vi "ClearDataContainer.vi"(8 "error in (no error)":errorcluster, 11 "Task_Abstr in":refnum<class "Task_Abstr.lvclass">) -> (0 "error out":errorcluster, 3 "Task_Abstr out":refnum<class "Task_Abstr.lvclass">)   [LabVIEW 2025, in "Task_Abstr.lvlib" / "Task_Abstr.lvclass"]
uses:
  Task_Abstr.lvclass
  DataContainer.ctl
  WaveformData.ctl
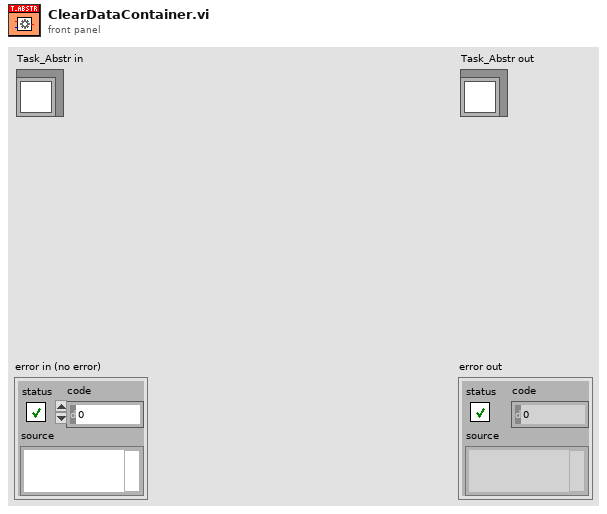
[diagram p1: front panel]
types:
  T1 = typedef "Task_Abstr.lvlib/Task_Abstr.lvclass/DataContainer.ctl" = map{string, T2}
  T2 = typedef "Task_Abstr.lvlib/Task_Abstr.lvclass/WaveformData.ctl" = cluster{"StartTime":timestamp, "StopTime":timestamp, "Waveform":waveform(dbl)[]}
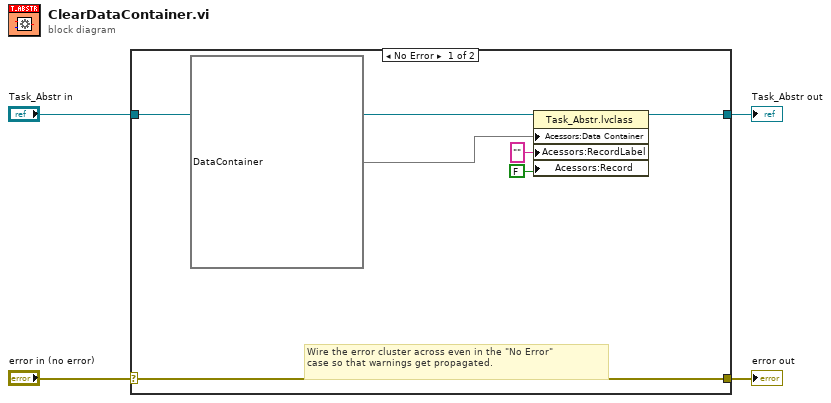
[diagram p0: block diagram]
diagram:
  n1 = case shown="No Error" "error in (no error)" {
    selector: "error in (no error)" -> [w9 w12]
    tunnel: [w9 w12] -> w3
    tunnel: [w8 w11] -> w1
    tunnel: "Task_Abstr in" -> [w10 w11]
    frame No Error {
      # "Wire the error cluster across even in the \"No Error\"\ncase so that warnings get propagated."
      n2 = property class="Task_Abstr.lvclass"(reference=w10, "Acessors:Data Container"=T1 {} ("Data Container"), "Acessors:RecordLabel"="" ("RecordLabel"), "Acessors:Record"=FALSE ("Record")) -> (reference out=w8:refnum<class "Task_Abstr.lvclass">)  [unwired: 1 in, 1 out]
    }
    frame Error {
    }
  }
  "error out" <- w3
  "Task_Abstr out" <- w1
